vi "Event handler-Ref laser power change.vi"(10 "Ref Laser Power":u8) -> ()   [LabVIEW 2017]
uses:
  Peripherals Control/Pockels/Globals/gl_Pockels control globals.vi
  Global Variables/gl_UI Ctrl Refs.vi
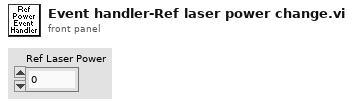
[diagram p1: front panel]
types:
  T1 = typedef "UI ctrl refs cluster.ctl" = cluster{"Top level VI path":path, "Top level VI ref":refnum<vi>, "User menu ref":refnum<k9>, "Sub Panel control":refnum<vi>, "Imaging Param Tab":refnum<vi>, "Occurrence-Start drivers":refnum<k4>, "Occurrence-Speed logging initialised":refnum<k4>, "Occurrence-XYZ stage initialised":refnum<k4>, "Exit button":refnum<vi>, "Status ind":refnum<vi>, "Set as origin":refnum<vi>, "Speed Logging":refnum<vi>, "Time Lapse":refnum<vi>, "Live Imaging":refnum<vi>, "AOL Z Stack":refnum<vi>, "Motor Z Stack":refnum<vi>, "Funct Acq button":refnum<vi>, "Hard Shutter":refnum<vi>, "Virtual Shutter":refnum<vi>, "Laser Power":refnum<vi>, "AOL Mode":refnum<vi>, "Frame Size":refnum<vi>, "Field of View":refnum<vi>, "Dwell Time":refnum<vi>, "Zoom":refnum<vi>, "AOL Z":refnum<vi>, "Objective":refnum<vi>, "Axis":refnum<vi>, "Paths & Names":refnum<vi>, "Experiment folder path (ind.)":refnum<vi>, "Last State (Ind.)":refnum<vi>, "Averages":refnum<vi>, "Angle (degrees)":refnum<vi>, "X centre":refnum<vi>, "Y centre":refnum<vi>, "Plane Mode":refnum<vi>, "# Planes":refnum<vi>, "Z Start":refnum<vi>, "Z Stop":refnum<vi>, "Z Step":refnum<vi>, "PMT 1":refnum<vi>, "PMT 2":refnum<vi>, "Stage XYZ Position":refnum<vi>, "Pockels@Z Start":refnum<vi>, "Pockels@Z Stop":refnum<vi>, "Obtain Z Start":refnum<vi>, "Obtain Z Stop":refnum<vi>, "Live stim.trig.period":refnum<vi>, "Live stim.trig.enable":refnum<vi>, "Movement Correction":refnum<vi>, "Load Reference Image":refnum<vi>, "XY Stage Move":refnum<vi>, "MovCor Cluster":refnum<vi>, "RefDAQParam":refnum<vi>, "Funct. Acq. Pockels Modulation":refnum<vi>, "Ref Laser Power":refnum<vi>, "Enable Video Recording":refnum<vi>, "Video Record-Live Imaging":refnum<vi>, "Video Record-Funct acq":refnum<vi>, "Reference Source":refnum<vi>, "AOL Z-stack Chirps Ready (ind)":refnum<vi>, "Target time between mov.cor. ref triggers (ms)":refnum<vi>, "Funct. Acq. Ref frame save":refnum<vi>, "Tracking button":refnum<vi>, "Show ref plots window":refnum<vi>, "Center freq ind (nm)":refnum<vi>, "Pickup mode (ind)":refnum<vi>, "Logging queue (ind)":refnum<vi>, "Back aperture power (ind.)":refnum<vi>, "Power after objective (ind.)":refnum<vi>, "Switch user":refnum<vi>, "Ls1 Conn. Status":refnum<vi>, "Ls1Tuning Status":refnum<vi>, "Ls1 Faults":refnum<vi>, "Ls1 Connection":refnum<vi>, "Ls1 Mode":refnum<vi>, "Ls1 POWER [mW]":refnum<vi>, "Ls1Shutter":refnum<vi>, "Ls1 Wavelength":refnum<vi>, "Ls1 Note":refnum<vi>, "Ls1 Confirm Wav":refnum<vi>, "Ls1 PreChrp Prism1":refnum<vi>, "Ls1 PreChrp Prism2":refnum<vi>, "Ls1 wav top Ind":refnum<vi>, "Ls1 power top Ind":refnum<vi>, "Ls1 Pump peak Hold":refnum<vi>, "Ls1 Status Ind":refnum<vi>, "Ls1 wav cancel":refnum<vi>, "Experiment Type":refnum<vi>, "Biology Information":refnum<vi>}
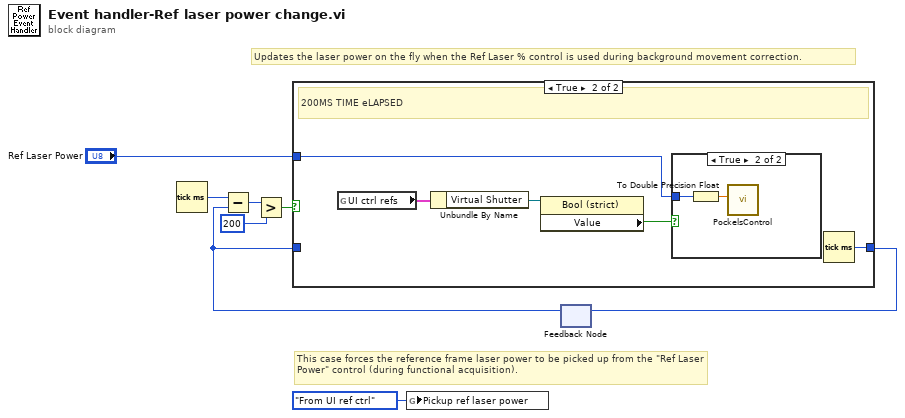
[diagram p0: block diagram]
diagram:
  # "This case forces the reference frame laser power to be picked up from the \"Ref Laser Power\" control (during functional acquisition)."
  # "Updates the laser power on the fly when the Ref Laser % control is used during background movement correction."
  n1 = Tick Count (ms)() -> (millisecond timer value=w2:u32)
  n2 = global write "gl_Pockels control globals.vi" "Pickup ref laser power"(enum16{"From source image", "From UI ref ctrl"}."From UI ref ctrl" ("Pickup ref laser power")) -> ()
  n3 = feedback #1() -> (w6:u32)  [unwired: 1 in]
  n4 = Subtract(x=w2, y=w6) -> (x-y=w3:u32)
  n5 = Greater?(x=w3, y=u32 200) -> (0:w5:bool)
  n6 = case shown="True" w5 {
    tunnel: "Ref Laser Power" -> [_ w11]
    tunnel: [w9 w14] -> w1
    tunnel: w6 -> [w9 _]
    frame False {
    }
    frame True {
      # "200MS TIME eLAPSED"
      n7 = global read "gl_UI Ctrl Refs.vi" "UI ctrl refs"() -> (w10:T1)
      n8 = Unbundle By Name(w10) -> ("Virtual Shutter"=w13:refnum<vi>)
      n9 = property class="Bool (strict)"(reference=w13) -> ("Value"=w12:bool)  [unwired: 1 in, 2 out]
      n10 = case shown="True" w12 {
        tunnel: w11 -> [_ w16]
        frame False {
        }
        frame True {
          n11 = To Double Precision Float(number=w16) -> (double precision float=w15:dbl)
          n12 = call "PockelsControl.vi"("Laser Power (%)"=w15) -> ()  [unwired: 10 in, 1 out]
        }
      }
      n13 = Tick Count (ms)() -> (millisecond timer value=w14:u32)
    }
  }
  n14 = feedback-in #1(w1) -> ()
